vi "DFD Build Filter Bank from Filter Coefficients.vi"(6 "fs in [Hz]":dbl=1.0, 8 "error in (no error)":errorcluster, 10 "band counts":i32=4, 11 "h(n)":dbl[](array[numeric])) -> (0 "error out":errorcluster, 3 "filter bank out":T1 {"mFBank_SynthesisFilters"."mMRate_SumWl" min=1 max=32 step=1; "mFBank_SynthesisFilters"."mMRate_InputIwl" min=1 max=32 step=1; "mFBank_SynthesisFilters"."mMRate_GainWl" min=1 max=32 step=1; "mFBank_SynthesisFilters"."mMRate_OutputWl" min=1 max=32 step=1; "mFBank_SynthesisFilters"."mMRate_InputWl" min=1 max=32 step=1; "mFBank_SynthesisFilters"."mMRate_CoefWl" min=1 max=32 step=1; "mFBank_SynthesisFilters"."mMRate_Mode" items=["Default"=-1, "No Rate Change"=0, "Interpolation"=1, "Decimation"=2, "Interpolated"=3, "Rational"=4]; "mFBank_AnalysisFilters"."mMRate_SumWl" min=1 max=32 step=1; "mFBank_AnalysisFilters"."mMRate_InputIwl" min=1 max=32 step=1; "mFBank_AnalysisFilters"."mMRate_GainWl" min=1 max=32 step=1; "mFBank_AnalysisFilters"."mMRate_OutputWl" min=1 max=32 step=1; "mFBank_AnalysisFilters"."mMRate_InputWl" min=1 max=32 step=1; "mFBank_AnalysisFilters"."mMRate_CoefWl" min=1 max=32 step=1; "mFBank_AnalysisFilters"."mMRate_Mode" items=["Default"=-1, "No Rate Change"=0, "Interpolation"=1, "Decimation"=2, "Interpolated"=3, "Rational"=4]; "mFBank_Type" items=["Uniform", "Non-Uniform"]})   [LabVIEW 2017, in "NI_DigFilter_FilterBank.lvlib"]
doc: "Creates a cosine-modulated filter bank from a prototype filter."
uses:
  <vilib>/addons/Digital Filter Design/NI_DigFilter_FilterBank.lvlib
  <vilib>/addons/Digital Filter Design/FilterBank.llb/Object/DFD Filter Bank Obj.ctl
  <vilib>/addons/Digital Filter Design/_Objects.llb/DFD Multirate Filter Obj.ctl
  <vilib>/addons/Digital Filter Design/_Objects.llb/DFD Multirate Mode.ctl
  <vilib>/addons/Digital Filter Design/_Objects.llb/DFD Coef Norm Type.ctl
  <vilib>/addons/Digital Filter Design/_Objects.llb/DFD Round-off Mode.ctl
  <vilib>/addons/Digital Filter Design/_Objects.llb/DFD FXP MRate Multiply Mode.ctl
  <vilib>/addons/Digital Filter Design/FilterBank.llb/Object/DFD Filter Bank Processing Method.ctl
  <vilib>/addons/Digital Filter Design/FilterBank.llb/Object/DFD Filter Bank Type.ctl
  <vilib>/addons/Digital Filter Design/NI_DigFilterLicensed.lvlib
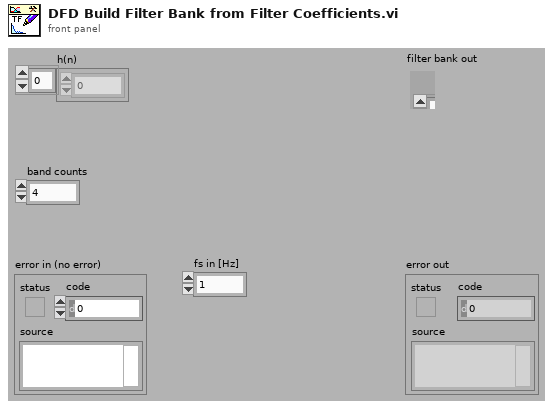
[diagram p1: front panel]
types:
  T1 = typedef "NI_DigFilter_FilterBank.lvlib/DFD Filter Bank Obj.ctl" = cluster{"mFBank_AnalysisFilters":T2[], "mFBank_SynthesisFilters":T2[], "mFBank_#Bands":i32, "mFBank_ProcMethod":T7, "mFBank_Coeffs":dbl[], "mFBank_Gain":dbl, "mFBank_Delay":i32, "mFBank_Type":T8}
  T2 = typedef "NI_DigFilterLicensed.lvlib/DFD Multirate Filter Obj.ctl" = cluster{"mMRate_Structure":enum16{"CIC", "FIR", "IIR", "Lattice"}, "mMRate_Mode":T3, "mMRate_Factor":i32, "mMRate_FIRParams":cluster{"mMRate_FIR_H":dbl[], "mMRate_FIR_IsNyquist?":bool, "mMRate_FIR_IsSymmetric?":bool}, "mMRate_CICParams":cluster{"mMRate_CIC_#Stage":i32, "mMRate_CIC_Lag":i32, "mMRate_CIC_Type":enum16{"Lowpass", "Highpass"}}, "mMRate_Order":i32, "mMRate_Version":string, "mMRate_Comments":string, "mMRate_RationalFactor":cluster{"mMRate_L":i32, "mMRate_M":i32}, "mMRate_Fs":dbl, "mMRate_Quantized?":bool, "mMRate_QFilterGain":dbl, "mMRate_CoefWl":i16, "mMRate_Scaling":cluster{"mMRate_ScaleByPowerOf2?":bool, "mMRate_ScaleType":T4}, "mMRate_InputWl":i16, "mMRate_OutputWl":i16, "mMRate_OutputMode":T5, "mMRate_MultMode":T6, "mMRate_BitPruning":bool, "mMRate_GainWl":i16, "mMRate_OutputFwl":i16, "mMRate_SumIwl":i16, "mMRate_InputIwl ":i16, "mMRate_SumWl":i16, "mMRate_CoefIwl":i16}
  T3 = typedef "NI_DigFilterLicensed.lvlib/DFD Multirate Mode.ctl" = i16
  T4 = typedef "NI_DigFilterLicensed.lvlib/DFD Coef Norm Type.ctl" = enum16{"No Norm", "Time Domain 1-Norm", "Time Domain 2-Norm", "Time Domain Inf-Norm"}
  T5 = typedef "NI_DigFilterLicensed.lvlib/DFD Round-off Mode.ctl" = enum16{"Nearest", "Truncation"}
  T6 = typedef "NI_DigFilterLicensed.lvlib/DFD FXP MRate Multiply Mode.ctl" = enum16{"Truncated", "Full"}
  T7 = typedef "NI_DigFilter_FilterBank.lvlib/DFD Filter Bank Processing Method.ctl" = enum16{"General", "2-Band QMF Lattice", "Cosine-Modulated"}
  T8 = typedef "NI_DigFilter_FilterBank.lvlib/DFD Filter Bank Type.ctl" = u16
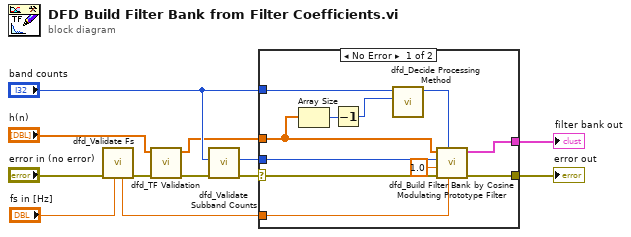
[diagram p0: block diagram]
diagram:
  n1 = call <vilib>:"dfd_Validate Fs.vi"("fs [Hz]"="fs in [Hz]", "error in (no error)"="error in (no error)") -> ("error out"=w3:errorcluster, "dup fs [Hz]"=w1:dbl)  [unwired: 8 in]
  n2 = call <vilib>:"dfd_TF Validation.vi"("error in (no error)"=w3, "numerator"="h(n)") -> ("error out"=w10:errorcluster, "validated numerator"=w6:dbl[])  [unwired: 1 in, 4 out]
  n3 = call <vilib>:"dfd_Validate Subband Counts.vi"("error in (no error)"=w10, "band counts"="band counts") -> ("error out"=w9:errorcluster, "dup band counts"=w5:i32)  [unwired: 8 in]
  n4 = case shown="No Error" w9 {
    selector: w9 -> [w14 w24]
    tunnel: "band counts" -> [w21 _]
    tunnel: [w17 w24] -> w12
    tunnel: w1 -> [w19 _]
    tunnel: [w18 _] -> w11
    tunnel: w6 -> [w16 _]
    tunnel: w5 -> [w15 _]
    frame No Error {
      n5 = Array Size(array=w16) -> (size(s)=w23:i32)
      n6 = Decrement(x=w23) -> (x-1=w22:i32)
      n7 = call <vilib>:"dfd_Decide Processing Method.vi"("order"=w22, "band counts"=w21) -> ("processing method"=w20:T7)  [unwired: 9 in]
      n8 = call <vilib>:"dfd_Build Filter Bank by Cosine Modulating Prototype Filter.vi"("fs in [Hz]"=w19, "processing method"=w20, "error in"=w14, "gain"=1.0, "band counts"=w15, "filter coefficients"=w16) -> ("error out"=w17:errorcluster, "filter bank out"=w18:T1)  [unwired: 4 in]
    }
    frame Error {
    }
  }
  "error out" <- w12
  "filter bank out" <- w11
